vi "Read Toolbox session.vi"(8 "error in (no error)":errorcluster, 11 "Toolbox in":refnum<class "Toolbox.lvclass">) -> (0 "error out":errorcluster, 2 "Toolbox session":T1={"client handle"=refnum, "URL out"="localhost:8012", "universe_id"=0, "devices_id"=[]}, 3 "Toolbox out":refnum<class "Toolbox.lvclass">)   [LabVIEW 2014, in "Driver_interaction.lvlib" / "Toolbox.lvclass"]
uses:
  Toolbox.lvclass
  Controls/Toolbox_session.ctl
  <vilib>/httpClient/ClientHandle.ctl
  Toolbox.lvclass/Toolbox.ctl
  <vilib>/httpClient/LabVIEWHTTPClient.lvlib
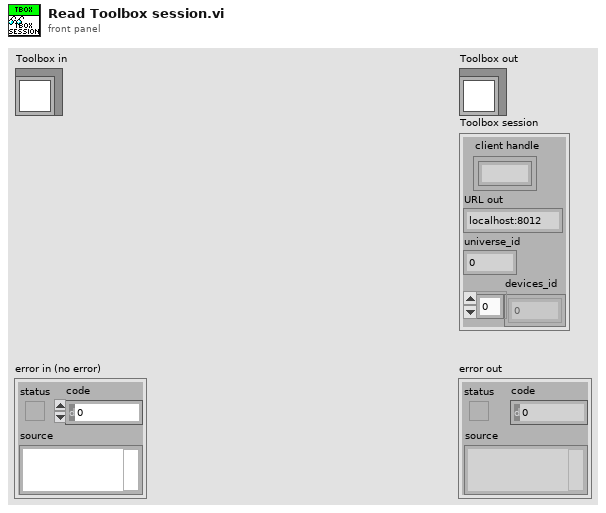
[diagram p1: front panel]
types:
  T1 = typedef "Driver_interaction.lvlib/Toolbox.lvclass/Toolbox_session.ctl" = cluster{"client handle":T2, "URL out":string, "universe_id":i32, "devices_id":i32[]}
  T2 = typedef "LabVIEWHTTPClient.lvlib/ClientHandle.ctl" = refnum<k1>
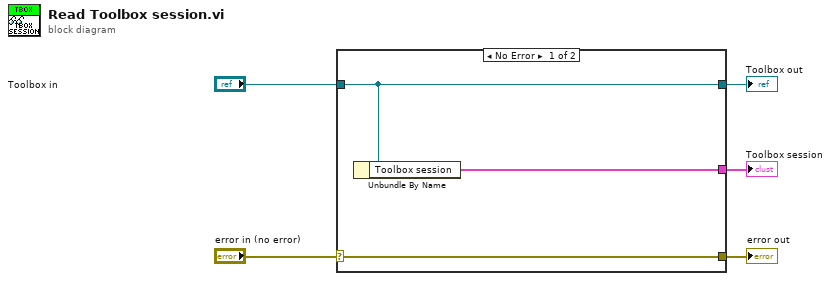
[diagram p0: block diagram]
diagram:
  n1 = case shown="No Error" "error in (no error)" {
    selector: "error in (no error)" -> [w8 w9]
    tunnel: [w8 w9] -> w4
    tunnel: [w7 w10] -> w2
    tunnel: "Toolbox in" -> [w7 w10]
    tunnel: [w6 _] -> w1
    frame No Error {
      n2 = Unbundle By Name(w7) -> ("Toolbox session"=w6:T1)
    }
    frame Error {
    }
  }
  "error out" <- w4
  "Toolbox out" <- w2
  "Toolbox session" <- w1
